vi "optionsAcq_gainOpticalDetector.vi"(0 "reference":refnum<class "OSA.lvclass">, 2 "gain_idx":u16=1, 4 "readWrite":enum16{"read", "write"}(ring), 5 "error in (no error)":errorcluster, 7 "ignore range violation (false)":bool) -> (14 "duplicate reference":refnum<class "OSA.lvclass">, 15 "status":string, 16 "gain_idx  out":u16, 17 "gain_relative":dbl, 19 "error out":errorcluster)   [LabVIEW 2010, in "OSA.lvclass"]
uses:
  OSA.lvclass
  _dll/LVLib/FTSLib.lvlib
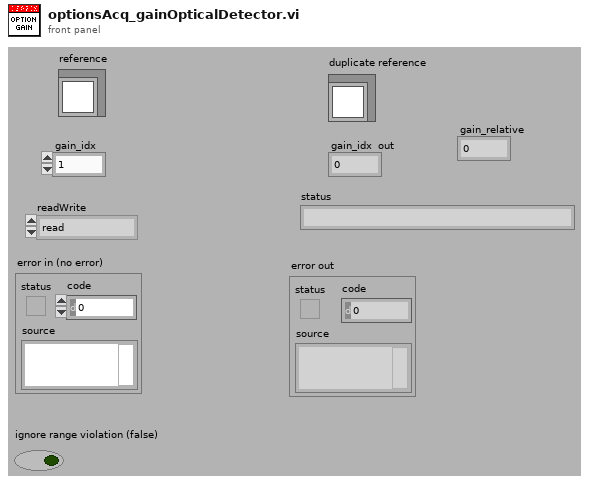
[diagram p1: front panel]
types:
  T1 = typedef "OSA.lvclass/ObjectAttributes.ctl" = cluster{"Stop":bool, "dataType":T2, "spectrometerIdx":u16, "buffer size interferogram":i32, "interferogram":cluster{"new":bool, "plot_x_ min":sgl, "plot_x_max":sgl, "plot_y_min":sgl, "plot_y_max":sgl, "Graph Intrfrgrm":T3, "timeStamp":u32, "signal (%)":dbl, "traces":cluster{"idx":u32, "broadBand":bool, "monoChromatic":bool, "peakToPeakSignal":dbl, "peakToPeakPos":dbl}[], "traces idx last":i32}, "spectrum":cluster{"new":bool, "plot_x_min":sgl, "plot_x_max":sgl, "plot_unit_x":T4, "plot_unit_y":T5, "plot_y_min":sgl, "plot_y_max":sgl, "Graph Spectrum":T3, "timeStamp":u32, "X_VAL_OPTIONS":enum16{"MIN_MAX", "ARRAY"}, "traces":cluster{"idx":u32}[], "traces idx last":i32}, "Thorlabs_OSA_64.lvclass:queue_action.ctlqueue ref":refnum<queue>, "action":T6, "plot zoom step":dbl, "buffer semaphore":T7, "acq stopped":bool, "dataType active":T2, "temperature (degr C)":sgl, "pressure (hPa)":sgl, "rel humidity (%)":sgl, "settings":cluster{"resolution":u16, "sensitivity":u16, "Average":bool, "average nr":u32, "apodisation":T8, "acq delay (ms)":u32, "airMesure":T9, "wmtr on":bool, "intfgrm_smooth_width":u16, "intfgrm_smooth_nrOfPasses":u16, "intfgrm_smooth":T10, "phaseCorrection":T11, "zeroFill":u8, "spectr_smooth":T10, "spectr_smooth_width":u16, "spectr_smooth_nrOfPasses":u16, "resolution (/cm)":sgl, "REF wavelength, (nm)":dbl, "gain_idx":u16, "gainAuto":bool, "gain_relative":dbl, "PD sensitivity mode":T12, "PD senseMode implemented":bool, "SensorTemperature implemented":bool, "SensorPressure implemented":bool, "SensorHumidity implemented":bool, "attenuationAuto":bool, "attenuationOnOff":bool, "attenuationAvailable":bool, "offsetAvailable":bool, "offset":i32, "offset max":u16}, "peaks position":sgl[], "peaks width":sgl[], "peaks height":sgl[], "peaks max nr":u32, "peaks latest nr":i32, "peaks new":bool, "power":dbl, "power new":bool, "path":string, "wavelength (WNr)":dbl, "wavelength new":bool, "buffer size spectrum":i32, "status":string, "VI reference":refnum<vi>, "funcPointer":u64, "libraryPointer":u64, "singleAcquisition":bool, "coherenceLength (cm)":dbl, "coherenceLength new":bool, "spectrometer model":string, "spectrometer serial nr":string, "peaks thld left":sgl[], "peaks thld right":sgl[], "coherenceLength error (cm)":dbl, "ADC bits":u16, "peaks position centroid":sgl[], "peaks height centroid":sgl[], "OSA series":T13, "channel index spectrum":u16, "spectrometer rangeLow, (/cm)":dbl, "spectrometer rangeHigh, (/cm)":dbl, "channel index interferogram":u16}
  T2 = typedef "OSA.lvclass/acq_dataType.ctl" = enum16{"none", "interferogram", "spectrum"}
  T3 = typedef "OSA.lvclass/graph_intensity.ctl" = refnum<vi>
  T4 = typedef "OSA.lvclass/spectrum_x_unit.ctl" = enum16{"wavenr/cm", "THz", "eV", "nm_air", "nm_vac"}
  T5 = typedef "OSA.lvclass/y_unit.ctl" = enum16{"ADC counts", "dBm pwr absolute", "dBm pwr density", "mW pwr absolute", "mW pwr density"}
  T6 = typedef "OSA.lvclass/queue_action.ctl" = enum16{"none", "stop", "GUI_plotInterferogram", "GUI_plotSpectrum", "GUI_plotInterferogramRescale", "GUI_plotSpectrumRescale", "GUI_plotInterferogramReset", "GUI_plotSpectrumReset", "GUI_plotInterferogramAutoScaleY", "GUI_plotSpectrumAutoScaleY", "GUI_plotInterferogramZoomOut", "GUI_plotSpectrumZoomOut", "GUI_plotInterferogramPane", "GUI_plotSpectrumPane", "GUI_plotInterferogramZoomMouse", "GUI_plotSpectrumZoomMouse", "GUI_spectrumChannelType", "GUI_channel", "ENVIRONMENT temperature", "ENVIRONMENT pressure", "MODE_resolution set", "MODE_resolution get", "MODE_sensitivity set", "MODE_sensitivity get", "MODE_PDTemperature set", "MODE_PDTemperature get", "REBOOT/RESET firmware", "ACQASYNC_acquireSingleSpectrum", "ACQASYNC_continuous start", "ACQASYNC_continuous stop\n", "ACQASYNC_get last interferogram", "ACQASYNC_get last spectrum", "ACQASYNC_get last waveNr", "ACQOPT_interferogram smoothing set", "ACQOPT_interferogram smoothing get", "ACQOPT_spectrum smoothing set", "ACQOPT_spectrum smoothing get", "ACQOPT_apodisation type set", "ACQOPT_apodisation type get", "ACQOPT_phase correction type set", "ACQOPT_phase correction type get", "ACQOPT_acqIntervall_set", "ACQOPT_acqIntervall_get", "ACQOPT_average spectrum set", "ACQOPT_average spectrum get", "ACQOPT_rolling average set", "ACQOPT_rolling average get", "ACQOPT_zero fill factor set", "ACQOPT_zero fill factor get", "ACQOPT_cycle counting set", "ACQOPT_cycle counting get", "ACQOPT_air measure option set", "ACQOPT_air measure option get", "ACQOPT_gainLevel auto get", "ACQOPT_gainLevel auto set", "ACQOPT_gainLevel get", "ACQOPT_gainLevel set", "ACQOPT_getAll", "INSTRUMENT_PROPERTY_range_WaveNr_min", "INSTRUMENT_PROPERTY_range_WaveNr_max", "INSTRUMENT_PROPERTY_reference_wavelength_cm^-1", "INSTRUMENT_PROPERTY_samplesPerRefPeriod", "INSTRUMENT_PROPERTY_resolution_waveNrPercm", "INSTRUMENT_PROPERTY_availableGainLevels", "INSTRUMENT_PROPERTY_status", "CONVERT", "ANALYSE_POWER", "ANALYSE_PEAKS", "ANALYSE_WAVELENGTH", "ANALYSE_SPECTRUM", "ANALYSE_INTERFEROGRAM", "ANALYSE_COHERENCE_LENGTH", "MATH", "MATH_power", "MATH_peaks", "FILE", "miscellaneous"}
  T7 = typedef "Semaphore RefNum" = refnum<k1>
  T8 = typedef "OSA.lvclass/apodisation.ctl" = enum16{"NONE", "NORTON_BEER_WEAK", "NORTON_BEER_MEDIUM", "NORTON_BEER_STRONG", "TRIANGULAR", "COSINE", "HANN", "HAMMING", "BLACKMANHARRIS3", "BLACKMANHARRIS4", "GAUSSIAN"}
  T9 = typedef "OSA.lvclass/airMeasure.ctl" = enum16{"TEMPERATURE", "PRESSURE"}
  T10 = typedef "OSA20X_misc.lvlib/interferogram_smoothing.ctl" = enum16{"NONE", "BINOMIAL", "SAVITSKY_GOLAY", "FOURIER", "MOVING_AVERAGE", "GAUSSIAN"}
  T11 = typedef "OSA.lvclass/phaseCorrection.ctl" = enum16{"NONE", "MERTZ", "FORMAN", "MERTZ_FILE", "FORMAN_FILE", "FUTURE COMP."}
  T12 = typedef "OSA20X_misc.lvlib/PDTemperatureMode.ctl" = enum16{"cool: better sensitivity/noise floor", "warm: extended wl range"}
  T13 = typedef "OSA.lvclass/OSA_series.ctl" = enum16{"OSA200", "OSA300", "UNKNOWN"}
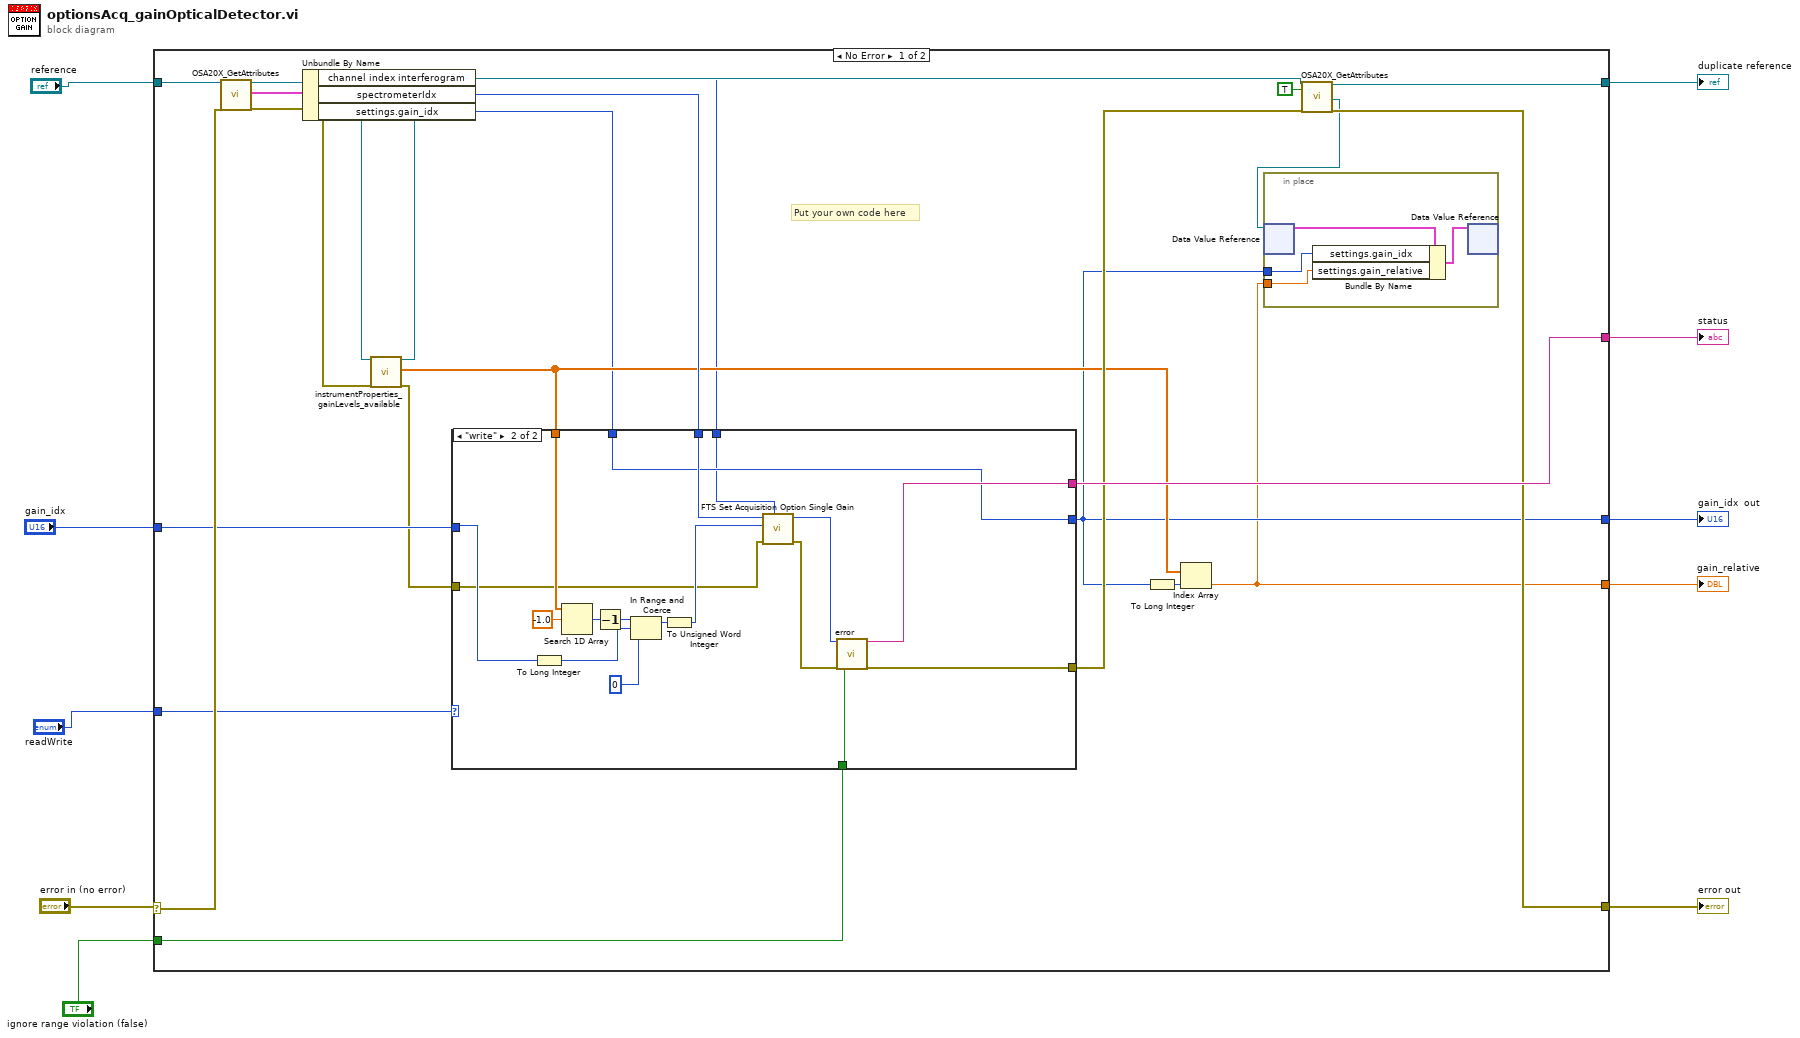
[diagram p0: block diagram]
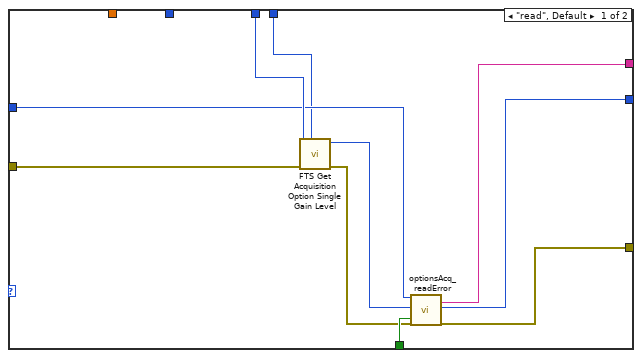
[diagram p2: hidden frame]
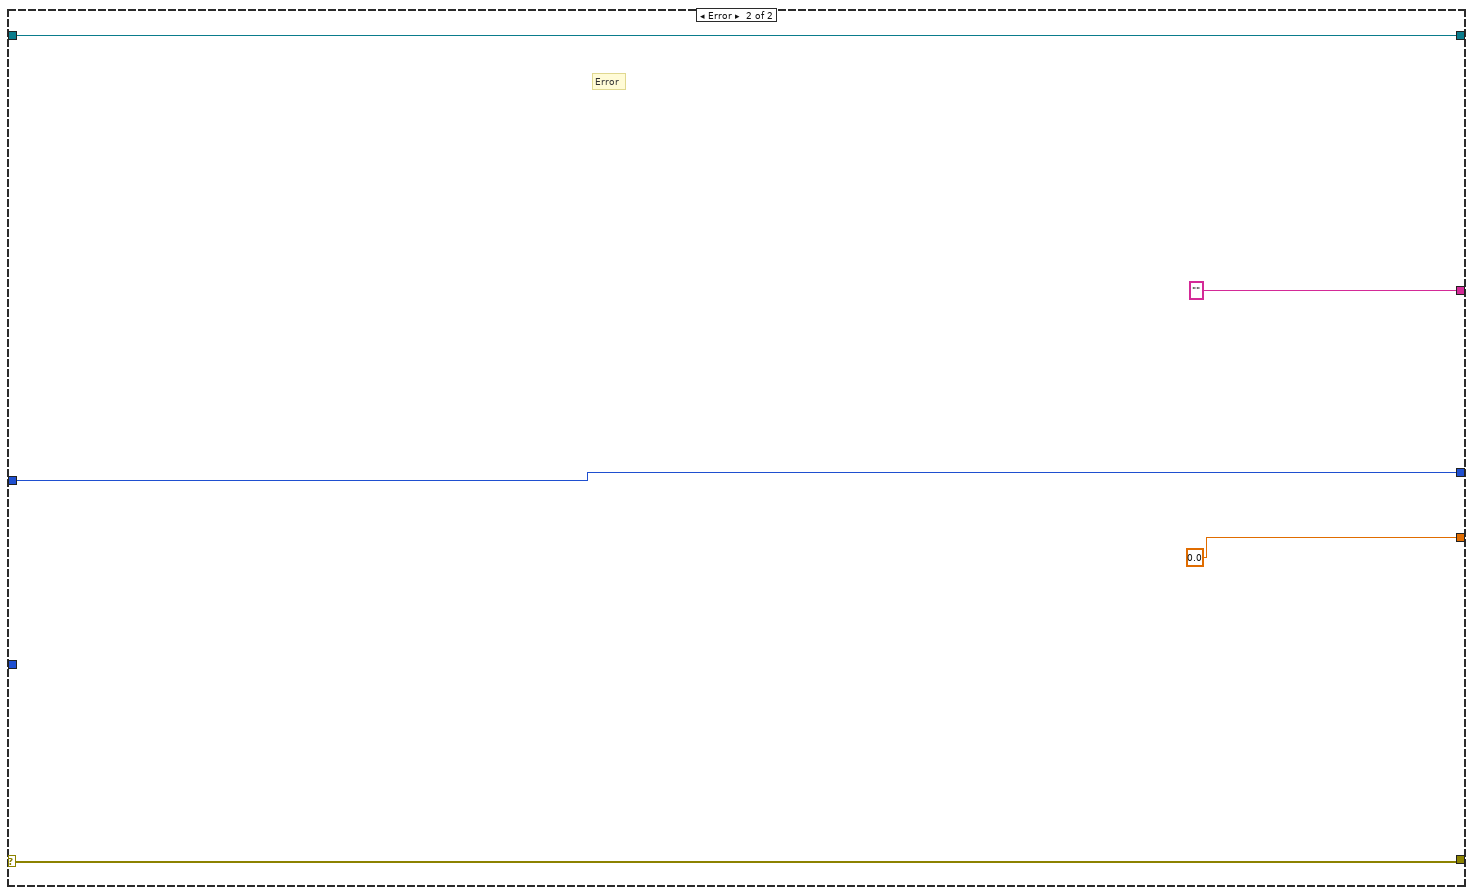
[diagram p3: hidden frame]
diagram:
  n1 = case shown="No Error" "error in (no error)" {
    selector: "error in (no error)" -> [w32 w69]
    tunnel: [w24 w69] -> w10
    tunnel: "reference" -> [w33 w70]
    tunnel: [w26 w70] -> w7
    tunnel: "readWrite" -> [w30 _]
    tunnel: "gain_idx" -> [w27 w67]
    tunnel: [w29 "" ("status")] -> w4
    tunnel: "ignore range violation (false)" -> [w28 _]
    tunnel: [w13 w67] -> w2
    tunnel: [w12 0.0 ("GainLevels 2")] -> w1
    frame No Error {
      # "Put your own code here"
      n2 = call "OSA20X_GetAttributes.vi"("reference in"=w33, "error in (no error)"=w32) -> ("reference out"=w23:refnum<class "OSA.lvclass">, "Data"=w15:T1, "error out"=w21:errorcluster)  [unwired: 14 in, 1 out]
      n3 = Unbundle By Name(w15) -> ("channel index interferogram"=w11:u16, "spectrometerIdx"=w31:u16, "settings.gain_idx"=w17:u16)
      n4 = call "instrumentProperties_gainLevels_available.vi"("reference"=w23, "error in (no error)"=w21) -> ("duplicate reference"=w22:refnum<class "OSA.lvclass">, "gainLevels out"=w19:dbl[], "error out"=w20:errorcluster)  [unwired: 15 in]
      n5 = case shown="\"write\"" w30 {
        tunnel: w31 -> [w44 w62]
        tunnel: w27 -> [w41 w56]
        tunnel: [w46 w64] -> w29
        tunnel: w28 -> [w47 w63]
        tunnel: [w39 w49] -> w13
        tunnel: [w45 w65] -> w25
        tunnel: w20 -> [w43 w51]
        tunnel: w19 -> [_ w52]
        tunnel: w17 -> [_ w49]
        tunnel: w11 -> [w38 w48]
        frame "read", Default {
          n6 = call "FTS Get Acquisition Option Single Gain Level.vi"("channel"=w38, "error in (no error)"=w43, "specIndex"=w44) -> ("error out"=w42:errorcluster, "function return"=w40:i32)  [unwired: 7 in]
          n7 = call "optionsAcq_readError.vi"("option default"=w41, "option return"=w40, "error in (no error)"=w42, "error ignore"=w47) -> ("status"=w46:string, "option"=w39:u16, "error out"=w45:errorcluster)  [unwired: 13 in]
        }
        frame "write" {
          n8 = To Long Integer(number=w56) -> (32bit integer=w55:i32)
          n9 = Search 1D Array(1D array=w52, element=-1.0) -> (index of element=w58:i32)  [unwired: 1 in]
          n10 = Decrement(x=w58) -> (x-1=w57:i32)
          n11 = In Range and Coerce(upper limit=w57, x=w55, lower limit=0) -> (coerced(x)=w54:i32)  [unwired: 1 out]
          n12 = To Unsigned Word Integer(number=w54) -> (unsigned 16bit integer=w53:u16)
          n13 = call "FTS Set Acquisition Option Single Gain.vi"("channel"=w48, "error in (no error)"=w51, "gainIndex"=w53, "specIndex"=w62) -> ("error out"=w60:errorcluster, "function return"=w61:i32)  [unwired: 6 in]
          n14 = call "error.vi"("result code"=w61, "error in (no error)"=w60, "ignore range violation"=w63) -> ("status"=w64:string, "error out"=w65:errorcluster)  [unwired: 14 in, 1 out]
        }
      }
      n15 = To Long Integer(number=w13) -> (32bit integer=w18:i32)
      n16 = Index Array(array=w19, index=w18) -> (element=w12:dbl)
      n17 = call "OSA20X_GetAttributes.vi"("reference in"=w22, "OnlyGetDvrReference(False)"=TRUE, "error in (no error)"=w25) -> ("reference out"=w26:refnum<class "OSA.lvclass">, "DataRef"=w14:refnum<data-value>, "error out"=w24:errorcluster)  [unwired: 13 in, 1 out]
      n18 = in-place {
        in-place-border: w13 -> [w36]
        in-place-border: w12 -> [w35]
        n19 = in-place-dvr #1(w14) -> (w37:T1)  [unwired: 1 out]
        n20 = Bundle By Name(cluster=w37, "settings.gain_idx"=w36, "settings.gain_relative"=w35) -> (w34:T1)
        n21 = in-place-dvr #1(w34) -> ()  [unwired: 2 out]
      }
    }
    frame Error {
      # "Error"
    }
  }
  "error out" <- w10
  "duplicate reference" <- w7
  "status" <- w4
  "gain_idx  out" <- w2
  "gain_relative" <- w1
